vi "view curr alr state_1.vi"(10 "ALR_Names":string[][](array[string]), 11 "ALR_State":T1) -> (1 "Ack_c":bool, 2 "N ack":i32, 3 "Ack":bool[](array[boolean]), 4 "n_alr":i32, 5 "This VI":refnum<vi>)   [LabVIEW 2019, in "Alarms.lvlib"]
uses:
  Alarms.lvlib
  Ctl/ALRs_State.ctl
  Logik/Logik.lvlib
panel:
  in  "Ack 6":bool
  in  "Ack 5":bool
  in  "Ack 4":bool
  in  "Ack 3":bool
  in  "Ack 2":bool
  in  "Ack 1":bool
  in  "n_elem":i32(c297)
  out "alr state 6":i32(ring)
  out "alr state 5":i32(ring)
  out "alr state 4":i32(ring)
  out "alr state 3":i32(ring)
  out "alr state 2":i32(ring)
  out "alr state 1":i32(ring)
  out "alrname 6":string
  out "alrname 5":string
  out "alrname 4":string
  out "alrname 3":string
  out "alrname 2":string
  out "alrname 1":string
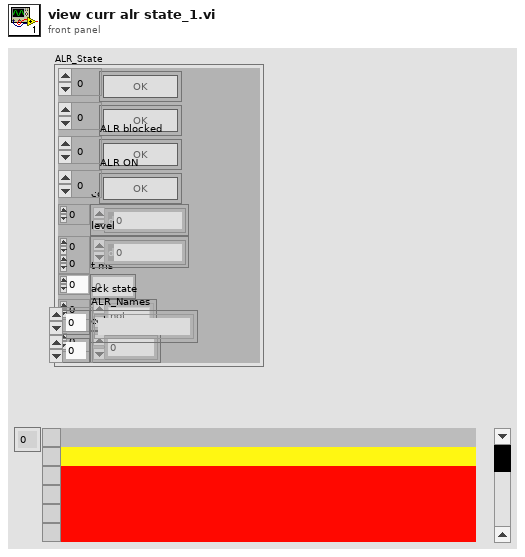
[diagram p1: front panel]
types:
  T1 = typedef "Alarms.lvlib/ALRs_State.ctl" = cluster{"ALR not block":bool[], "ALR":bool[], "ALR blocked":bool[], "ALR ON":bool[], "code":i32[], "level":i32[][], "t ms":u32[], "ack state":enum32{"not", "tripped", "reset", "ack"}[], "color":u32[]}
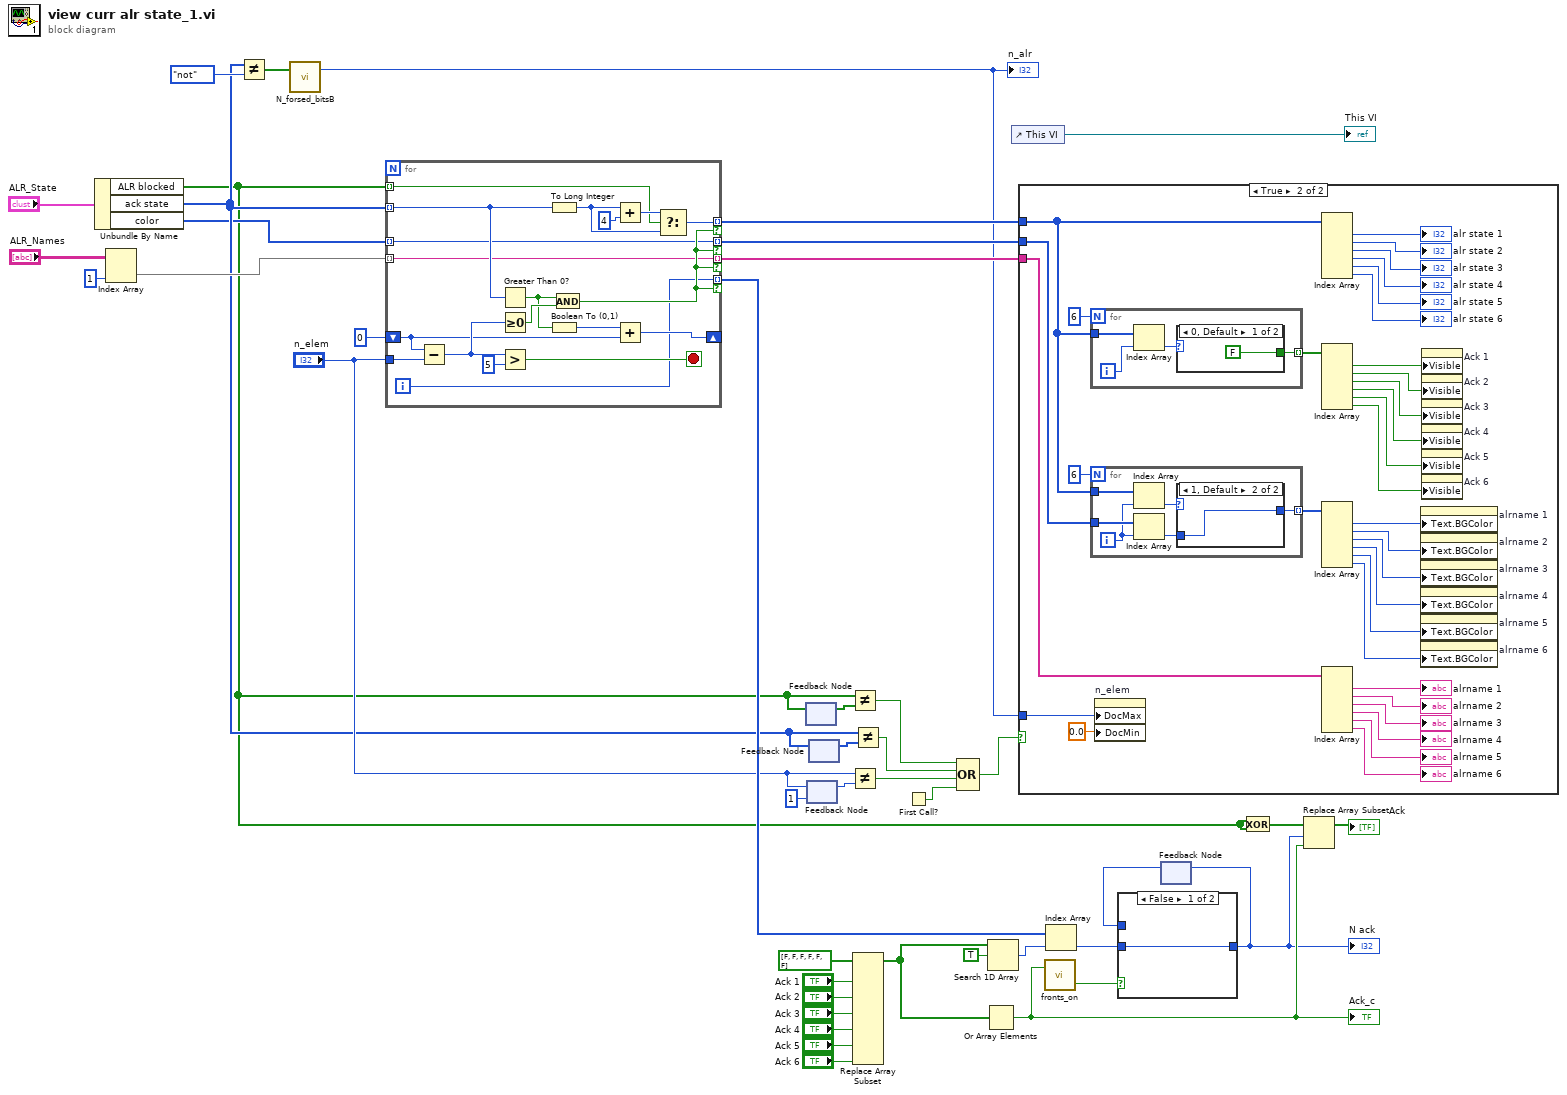
[diagram p0: block diagram]
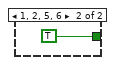
[diagram p4: hidden frame]
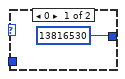
[diagram p5: hidden frame]
diagram:
  n1 = Unbundle By Name("ALR_State") -> ("ALR blocked"=w4:bool[], "ack state"=w6:enum32{"not", "tripped", "reset", "ack"}[], "color"=w5:u32[])
  n2 = Index Array(array="ALR_Names", index (col)=1 ("disabled index (col)")) -> (element=w13:string[])  [unwired: 1 in]
  n3 = Not Equal?(x=w6, y=enum32{"not", "tripped", "reset", "ack"}."not" ("ack state")) -> (x != y?=w10:bool[])
  n4 = call "N_forsed_bitsB.vi"("IN"=w10) -> ("N_forsed_bits"=w7:i32)  [unwired: 2 in]
  "n_alr" <- w7
  n5 = for {
    shift-right: [w61] -> _
    shift-left: 0 -> [w54]
    tunnel: [w60] -> w26 mode=indexing if=w50
    tunnel: [w47] -> w25 mode=indexing if=w50
    tunnel: [w46] -> w41 mode=indexing if=w50
    tunnel: [w45] -> w40 mode=indexing if=w50
    tunnel: "n_elem" -> [w53]
    tunnel: w6 -> [w48] mode=indexing
    tunnel: w5 -> [w47] mode=indexing
    tunnel: w13 -> [w46] mode=indexing
    tunnel: w4 -> [w44] mode=indexing
    i -> [w45]
    stop <- w49 stop-if-true
    n6 = Subtract(x=w54, y=w53) -> (x-y=w55:i32)
    n7 = Greater Than 0?(x=w48) -> (x > 0?=w51:bool)
    n8 = Greater Or Equal To 0?(x=w55) -> (x >= 0?=w52:bool)
    n9 = Greater?(x=w55, y=5) -> (0:w49:bool)
    n10 = To Long Integer(number=w48) -> (32bit integer=w57:i32)
    n11 = Boolean To (0,1)(Boolean=w51) -> (0, 1=w62:i16)
    n12 = And(x=w51, y=w52) -> (x .and. y?=w50:bool)
    n13 = Add(x=w57, y=4) -> (x+y=w58:i32)
    n14 = Add(x=w62, y=w54) -> (x+y=w61:i32)
    n15 = Select(t=w58, s=w44, f=w57) -> (s? t:f=w60:i32)
  }
  n16 = feedback #1() -> (w11:bool[])  [unwired: 1 in]
  n17 = feedback-in #1(w4) -> ()
  n18 = feedback #2(1 ("n_elem")) -> (w28:i32)
  n19 = feedback-in #2("n_elem") -> ()
  n20 = feedback #3() -> (w12:enum32{"not", "tripped", "reset", "ack"}[])  [unwired: 1 in]
  n21 = feedback-in #3(w6) -> ()
  n22 = Not Equal?(x=w4, y=w11) -> (x != y?=w1:bool)
  n23 = Not Equal?(x="n_elem", y=w28) -> (x != y?=w21:bool)
  n24 = Not Equal?(x=w6, y=w12) -> (x != y?=w2:bool)
  n25 = Replace Array Subset(array=bool[] [FALSE, FALSE, FALSE, FALSE, FALSE, FALSE], new element #1="Ack 1", new element #2="Ack 2", new element #3="Ack 3", new element #4="Ack 4", new element #5="Ack 5", new element #6="Ack 6") -> (w24:bool[])  [unwired: 6 in]
  n26 = First Call?() -> (First Call?: T/F=w3:bool)
  n27 = Compound Arithmetic op=OR(w1, w2, w21, w3) -> (w27:bool)
  n28 = Or Array Elements(Boolean array=w24) -> (logical OR=w20:bool)
  "Ack_c" <- w20
  n29 = Search 1D Array(1D array=w24, element=TRUE) -> (index of element=w22:i32)  [unwired: 1 in]
  n30 = control-ref of="This VI"() -> (→"This VI":refnum<vi>)
  n31 = case shown="True" w27 {
    tunnel: w41 -> [_ w71]
    tunnel: w26 -> [_ w67]
    tunnel: w25 -> [_ w66]
    tunnel: w7 -> [_ w63]
    frame False {
    }
    frame True {
      n32 = for {
        N: 6 -> [_]
        tunnel: w67 -> [w97]
        tunnel: [w99] -> w70 mode=indexing
        i -> [w98]
        n33 = Index Array(array=w97, index=w98) -> (element=w96:i32)
        n34 = case shown="0, Default" w96 {
          tunnel: [FALSE TRUE] -> w99
          frame 0, Default {
          }
          frame 1, 2, 5, 6 {
          }
        }
      }
      n35 = for {
        N: 6 -> [_]
        tunnel: w67 -> [w106]
        tunnel: [w107] -> w65 mode=indexing
        tunnel: w66 -> [w104]
        i -> [w103]
        n36 = Index Array(array=w106, index=w103) -> (element=w105:i32)
        n37 = Index Array(array=w104, index=w103) -> (element=w102:u32)
        n38 = case shown="1, Default" w105 {
          tunnel: [13816530 ("color") w109] -> w107
          tunnel: w102 -> [_ w109]
          frame 0 {
          }
          frame 1, Default {
          }
        }
      }
      n39 = property on="n_elem" class="Scroll (strict)"("DocMax"=w63, "DocMin"=0.0 ("Data Entry Limits:Minimum")) -> ()  [unwired: 2 in, 2 out]
      n40 = Index Array(array=w67) -> (element #1=→"alr state 1":i32, element #2=→"alr state 2":i32, element #3=→"alr state 3":i32, element #4=→"alr state 4":i32, element #5=→"alr state 5":i32, element #6=→"alr state 6":i32)  [unwired: 6 in]
      n41 = Index Array(array=w70) -> (element #1=w77:bool, element #2=w76:bool, element #3=w75:bool, element #4=w74:bool, element #5=w73:bool, element #6=w72:bool)  [unwired: 6 in]
      n42 = Index Array(array=w65) -> (element #1=w86:u32, element #2=w90:u32, element #3=w89:u32, element #4=w88:u32, element #5=w87:u32, element #6=w84:u32)  [unwired: 6 in]
      n43 = Index Array(array=w71) -> (element #1=→"alrname 1":string, element #2=→"alrname 2":string, element #3=→"alrname 3":string, element #4=→"alrname 4":string, element #5=→"alrname 5":string, element #6=→"alrname 6":string)  [unwired: 6 in]
      n44 = property on="alrname 1" class="Str"("Text.BGColor"=w86) -> ()  [unwired: 2 in, 2 out]
      n45 = property on="alrname 2" class="Str"("Text.BGColor"=w90) -> ()  [unwired: 2 in, 2 out]
      n46 = property on="alrname 3" class="Str"("Text.BGColor"=w89) -> ()  [unwired: 2 in, 2 out]
      n47 = property on="alrname 4" class="Str"("Text.BGColor"=w88) -> ()  [unwired: 2 in, 2 out]
      n48 = property on="alrname 5" class="Str"("Text.BGColor"=w87) -> ()  [unwired: 2 in, 2 out]
      n49 = property on="alrname 6" class="Str"("Text.BGColor"=w84) -> ()  [unwired: 2 in, 2 out]
      n50 = property on="Ack 1" class="Bool"("Visible"=w77) -> ()  [unwired: 2 in, 2 out]
      n51 = property on="Ack 2" class="Bool"("Visible"=w76) -> ()  [unwired: 2 in, 2 out]
      n52 = property on="Ack 3" class="Bool"("Visible"=w75) -> ()  [unwired: 2 in, 2 out]
      n53 = property on="Ack 4" class="Bool"("Visible"=w74) -> ()  [unwired: 2 in, 2 out]
      n54 = property on="Ack 5" class="Bool"("Visible"=w73) -> ()  [unwired: 2 in, 2 out]
      n55 = property on="Ack 6" class="Bool"("Visible"=w72) -> ()  [unwired: 2 in, 2 out]
    }
  }
  n56 = call "fronts_on.vi"("in"=w20) -> ("fall"=w18:bool)  [unwired: 1 in, 1 out]
  n57 = Index Array(array=w40, index=w22) -> (element=w19:i32)
  n58 = feedback #4() -> (w17:i32)  [unwired: 1 in]
  n59 = case shown="False" w18 {
    tunnel: w19 -> [w110 _]
    tunnel: [w110 w111] -> w16
    tunnel: w17 -> [_ w111]
    frame False {
    }
    frame True {
    }
  }
  "N ack" <- w16
  n60 = feedback-in #4(w16) -> ()
  n61 = Exclusive Or(1:w4, 2:w4) -> (0:w32:bool[])
  n62 = Replace Array Subset(array=w32, new element=w20, index=w16) -> (→"Ack":bool[])
